vi "Send Write Single Calibration Curve to Instrument.vi"(7 "Message Priority (Normal)":T1=enum."Normal", 8 "error in (no error)":errorcluster, 9 "Channel":i32, 10 "Calibration File":path, 11 "Message Enqueuer":refnum<class "Message Enqueuer.lvclass">) -> (0 "error out":errorcluster, 3 "Message Enqueuer out":refnum<class "Message Enqueuer.lvclass">)   [LabVIEW 2016, in "LS218.lvlib" / "Write Single Calibration Curve to Instrument Msg.lvclass"]
doc: "Sends the <B>LS218.lvlib:Write Single Calibration Curve to Instrument Msg.lvclass</B> message.\n\n<B>LS218.lvlib:LS218.lvclass:Write Single Calibration Curve to Instrument.vi</B> Description:\n\nRead one calibration curve from file and write to instrument (user calibration 21-28)."
uses:
  Write Single Calibration Curve to Instrument Msg.lvclass
  <vilib>/ActorFramework/Message Enqueuer/Message Enqueuer.lvclass
  <vilib>/ActorFramework/Message Enqueuer/Message Priority.ctl
  C:/Program Files (x86)/National Instruments/LabVIEW 2016/vi.lib/ActorFramework/Message/Message.lvclass
  Write Single Calibration Curve to Instrument Msg.lvclass/Write Single Calibration Curve to Instrument Msg.ctl
  <vilib>/ActorFramework/Message Enqueuer/Message Enqueuer.lvclass/Message Enqueuer.ctl
  <vilib>/ActorFramework/Message Priority Queue/Priority Enqueue.vi
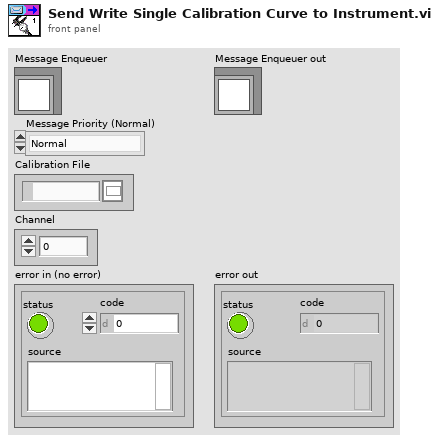
[diagram p1: front panel]
types:
  T1 = typedef "Actor Framework.lvlib/Message Enqueuer.lvclass/Message Priority.ctl" = enum16{"Low", "Normal", "High"}
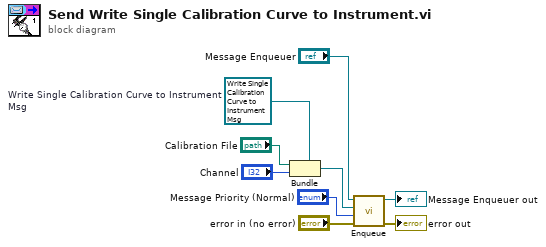
[diagram p0: block diagram]
diagram:
  w3 = refnum<class "Write Single Calibration Curve to Instrument Msg.lvclass"> refnum  # Write Single Calibration Curve to Instrument Msg
  n1 = Bundle(cluster=w3, "Calibration File", "Channel") -> (w6:refnum<class "Write Single Calibration Curve to Instrument Msg.lvclass">)
  n2 = call <vilib>:"Enqueue.vi"("error in (no error)"="error in (no error)", "Message Priority (Normal)"="Message Priority (Normal)", "Message"=w6, "Message Enqueuer in"="Message Enqueuer") -> ("error out"=→"error out":errorcluster, "Message Enqueuer out"=→"Message Enqueuer out":refnum<class "Message Enqueuer.lvclass">)  [unwired: 6 in]
